vi "Verify Font availability.vi"(5 "System Fonts":T1, 7 "Font name":string, 9 "One button message (F)?":bool, 11 "error in (no error)":errorcluster) -> (8 "Font":string, 15 "error out":errorcluster)   [LabVIEW 2013]
doc: "Version 1.0\nDeveloped by Jean-Marc Simard\nCopyright © 2010, Exaprom Inc.\nAll rights reserved.\nLicense: BSD\n\nWith iTextSharp 4.1.6 (http://itextsharp.sourceforge.net)\nunder Mozilla Public License Version 1.1\n(http://www.mozilla.org/MPL/MPL-1.1.html)"
uses:
  Controls/System Fonts.ctl
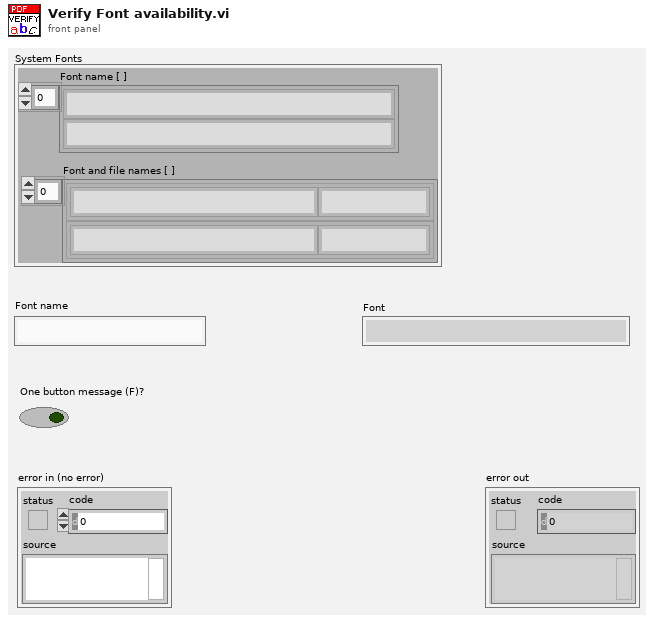
[diagram p1: front panel]
types:
  T1 = typedef "System Fonts.ctl" = cluster{"Font name [ ]":string[], "Font and file names [ ]":cluster{"Font name":string, "File name":string}[]}
  T2 = cluster{"Font name":string, "File name":string}[]
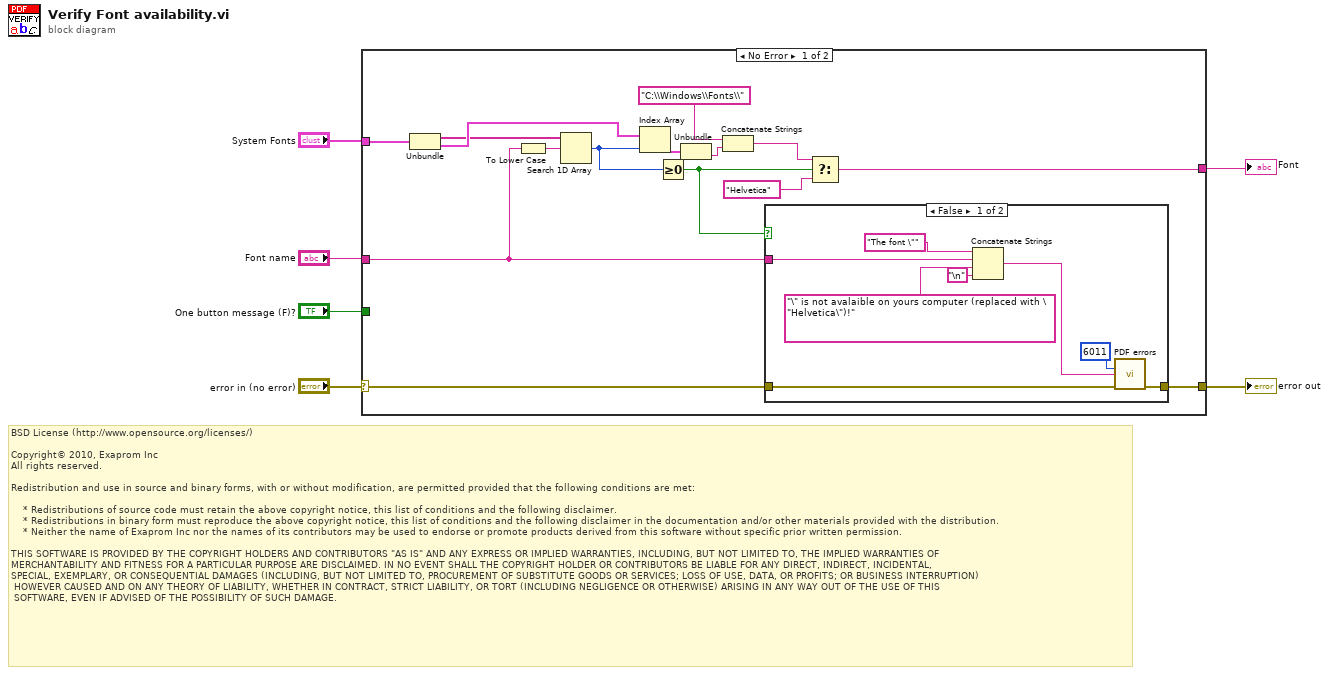
[diagram p0: block diagram]
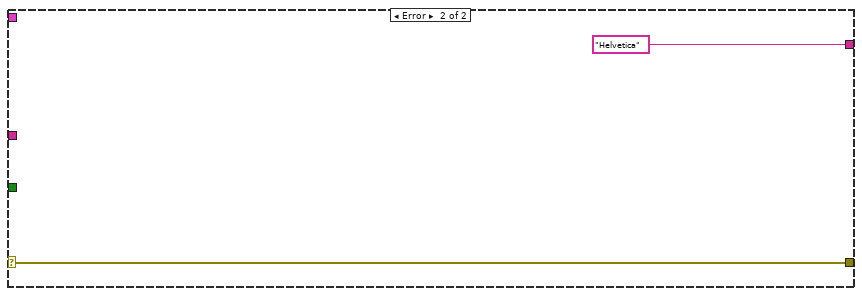
[diagram p3: hidden frame]
diagram:
  # "BSD License (http://www.opensource.org/licenses/)\n\nCopyright© 2010, Exaprom Inc\nAll rights reserved.\n\nRedistribution and use in source and binary forms, with or without modification, are permitted provided that the following conditions are met:\n\n    * Redistributions of source code must retain the above copyright notice, this list of conditions and the following disclaimer.\n    * Redistributions in binary form must reproduce the above copyright notice, this list of conditions and the following disclaimer in the documentation and/or other materials provided with the distribution.\n    * Neither the name of Exaprom Inc nor the names of its contributors may be used to endorse or promote products derived from this software without specific prior written permission.\n\nTHIS SOFTWARE IS PROVIDED BY THE COPYRIGHT HOLDERS AND CONTRIBUTORS \"AS IS\" AND ANY EXPRESS OR IMPLIED WARRANTIES, INCLUDING, BUT NOT LIMITED TO, THE IMPLIED WARRANTIES OF \nMERCHANTABILITY AND FITNESS FOR A PARTICULAR PURPOSE ARE DISCLAIMED. IN NO EVENT SHALL THE COPYRIGHT HOLDER OR CONTRIBUTORS BE LIABLE FOR ANY DIRECT, INDIRECT, INCIDENTAL,\nSPECIAL, EXEMPLARY, OR CONSEQUENTIAL DAMAGES (INCLUDING, BUT NOT LIMITED TO, PROCUREMENT OF SUBSTITUTE GOODS OR SERVICES; LOSS OF USE, DATA, OR PROFITS; OR BUSINESS INTERRUPTION)\n HOWEVER CAUSED AND ON ANY THEORY OF LIABILITY, WHETHER IN CONTRACT, STRICT LIABILITY, OR TORT (INCLUDING NEGLIGENCE OR OTHERWISE) ARISING IN ANY WAY OUT OF THE USE OF THIS\n SOFTWARE, EVEN IF ADVISED OF THE POSSIBILITY OF SUCH DAMAGE."
  n1 = case shown="No Error" "error in (no error)" {
    selector: "error in (no error)" -> [w7 w32]
    tunnel: [w8 w32] -> w6
    tunnel: [w12 "Helvetica"] -> w4
    tunnel: "System Fonts" -> [w11 _]
    tunnel: "Font name" -> [w10 _]
    tunnel: "One button message (F)?" -> [_ _]
    frame No Error {
      n2 = Unbundle(w11) -> ("Font name [ ]"=w20:string[], "Font and file names [ ]"=w21:T2)
      n3 = To Lower Case(string=w10) -> (all lower case string=w19:string)
      n4 = Search 1D Array(1D array=w20, element=w19) -> (index of element=w16:i32)  [unwired: 1 out]
      n5 = Index Array(array=w21, index=w16) -> (element=w14:cluster{"Font name":string, "File name":string})
      n6 = Greater Or Equal To 0?(x=w16) -> (x >= 0?=w9:bool)
      n7 = Unbundle(w14) -> ("File name"=w15:string)  [unwired: 1 out]
      n8 = Concatenate Strings("C:\\Windows\\Fonts\\", w15) -> (w17:string)
      n9 = case shown="False" w9 {
        tunnel: w10 -> [w28 _]
        tunnel: [w25 w30] -> w8
        tunnel: w7 -> [w24 w30]
        frame False {
          n10 = Concatenate Strings("The font \"", w28, "\" is not avalaible on yours computer (replaced with \"Helvetica\")!" ("string"), "\n") -> (w23:string)
          n11 = call "PDF errors.vi"("code"=6011, "Additionnal information"=w23, "error in (no error)"=w24) -> ("error out"=w25:errorcluster)  [unwired: 12 out]
        }
        frame True {
        }
      }
      n12 = Select(t=w17, s=w9, f="Helvetica") -> (s? t:f=w12:string)
    }
    frame Error {
    }
  }
  "error out" <- w6
  "Font" <- w4
